vi "subXMLGetBuildSpecs.vi"(11 "Refnum in":refnum<k20>) -> (1 "Buid spec section":string, 3 "Nodes":refnum<k20>[](array[refnum]))   [LabVIEW 2019, in "SolutionBuilder.lvlib" / "SolutionBuilder.lvclass"]
uses:
  SolutionBuilder.lvclass
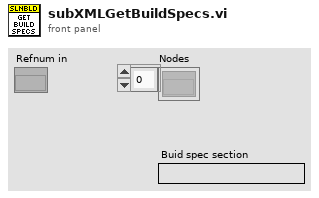
[diagram p1: front panel]
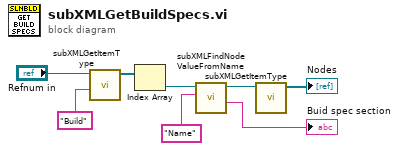
[diagram p0: block diagram]
diagram:
  n1 = call "subXMLGetItemType.vi"("Property value"="Build", "Refnum in"="Refnum in") -> ("Nodes"=w2:refnum<k20>[])  [unwired: 9 in]
  n2 = Index Array(array=w2) -> (element=w6:refnum<k20>)  [unwired: 1 in]
  n3 = call "subXMLFindNodeValueFromName.vi"("Property name"="Name", "Refnum in"=w6) -> ("Value"=→"Buid spec section":string, "Refnum out"=w7:refnum<k20>)  [unwired: 7 in, 1 out]
  n4 = call "subXMLGetItemType.vi"("Refnum in"=w7) -> ("Nodes"=→"Nodes":refnum<k20>[])  [unwired: 10 in]
